vi "remove no error text from control.vi"(11 "vis":refnum<vi>[](array[refnum])) -> (0 "error report":errorcluster[](array[cluster]))   [LabVIEW 2013, in "cosmetic changes.lvclass"]
uses:
  cosmetic changes.lvclass
  <vilib>/Utility/VariantDataType/VariantType.lvlib
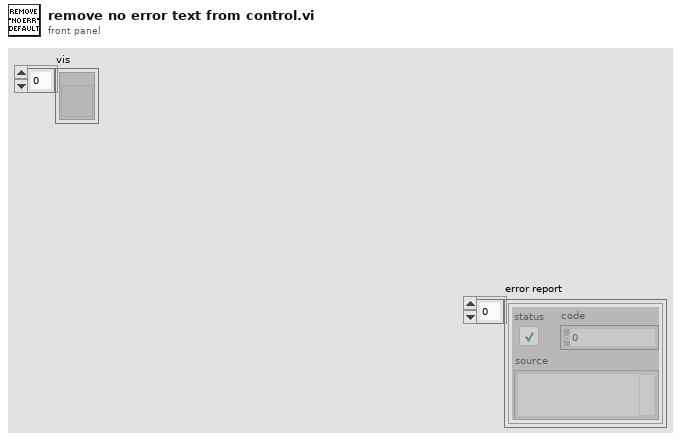
[diagram p1: front panel]
types:
  T1 = typedef "VariantType.lvlib/Type.ctl" = enum8{"Invalid Type", "Void", "I8", "I16", "I32", "I64", "U8", "U16", "U32", "U64", "Single Float", "Double Float", "Extended Float", "Single Complex", "Double Complex", "Extended Complex", "Enum U8", "Enum U16", "Enum U32", "Enum U64", "Single Float With Unit", "Double Float With Unit", "Extended Float With Unit", "Single Complex with Unit", "Double Complex with Unit", "Extended Complex with Unit", "Boolean", "String", "Path", "Picture", "Tag", "Array", "Cluster", "Variant", "LV Variant", "Waveform", "Timestamp", "Digital Waveform", "Digital Data", "ExpressData", "Refnum", "External Data", "VI", "Poly VI", "LabVIEW Class Instance", "Fixed Point"}
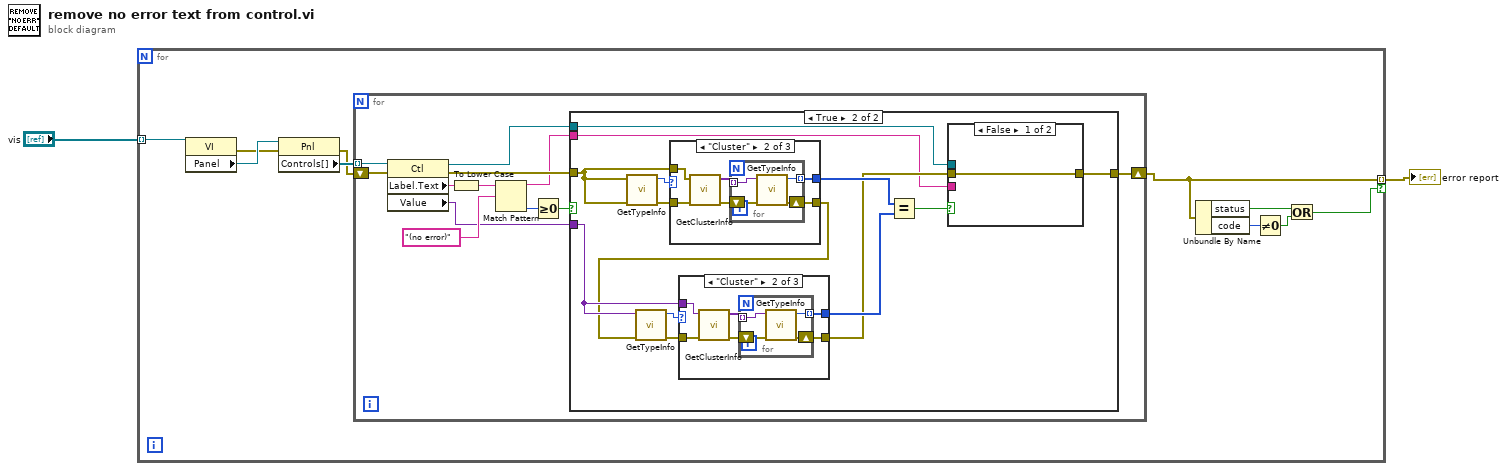
[diagram p0: block diagram]
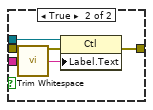
[diagram p3: hidden frame]
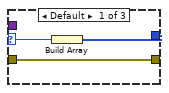
[diagram p4: hidden frame]
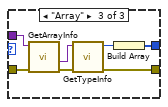
[diagram p5: hidden frame]
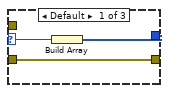
[diagram p6: hidden frame]
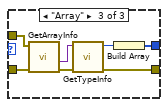
[diagram p7: hidden frame]
diagram:
  n1 = for {
    tunnel: "vis" -> [w8] mode=indexing
    tunnel: [w4] -> w1 mode=indexing if=w3
    n2 = property class="VI"(reference=w8) -> (error out=w11:errorcluster, "Panel"=w12:refnum<vi>)  [unwired: 1 in, 1 out]
    n3 = property class="Pnl"(reference=w12, error in=w11) -> (error out=w9:errorcluster, "Controls[]"=w10:refnum<vi>[])  [unwired: 1 out]
    n4 = for {
      tunnel: w10 -> [w24] mode=indexing
      shift-right: [w15] -> w4
      shift-left: w9 -> [w23]
      n5 = property class="Ctl"(reference=w24, error in=w23) -> (reference out=w14:refnum<vi>, error out=w16:errorcluster, "Label.Text"=w22:string, "Value"=w17:variant)
      n6 = To Lower Case(string=w22) -> (all lower case string=w21:string)
      n7 = Match Pattern(string=w21, regular expression="(no error)") -> (before substring=w13:string, offset past match=w19:i32)  [unwired: 1 in, 2 out]
      n8 = Greater Or Equal To 0?(x=w19) -> (x >= 0?=w18:bool)
      n9 = case shown="True" w18 {
        tunnel: w17 -> [_ w34]
        tunnel: w16 -> [w25 w37]
        tunnel: [w25 w29] -> w15
        tunnel: w14 -> [_ w28]
        tunnel: w13 -> [_ w27]
        frame False {
        }
        frame True {
          n10 = call <vilib>:"GetTypeInfo.vi"("error in (no error)"=w37, "Variant"=w37) -> ("error out"=w38:errorcluster, "Type Enum"=w39:T1)  [unwired: 5 in, 3 out]
          n11 = case shown="\"Cluster\"" w39 {
            selector: w39 -> [w68 _ _]
            tunnel: w37 -> [_ w74 w85]
            tunnel: [w67 w72 w82] -> w32
            tunnel: w38 -> [w66 w71 w80]
            tunnel: [w66 w69 w79] -> w33
            frame Default {
              n12 = Build Array(w68) -> (w67:T1[])
            }
            frame "Cluster" {
              n13 = call <vilib>:"GetClusterInfo.vi"("error in (no error)"=w71, "Variant"=w74) -> ("error out"=w70:errorcluster, "Cluster Elements"=w73:variant[])  [unwired: 8 in]
              n14 = for {
                tunnel: w73 -> [w78] mode=indexing
                tunnel: [w77] -> w72 mode=indexing
                shift-right: [w76] -> w69
                shift-left: w70 -> [w75]
                n15 = call <vilib>:"GetTypeInfo.vi"("error in (no error)"=w75, "Variant"=w78) -> ("error out"=w76:errorcluster, "Type Enum"=w77:T1)  [unwired: 5 in, 3 out]
              }
            }
            frame "Array" {
              n16 = call <vilib>:"GetArrayInfo.vi"("error in (no error)"=w80, "Variant"=w85) -> ("error out"=w81:errorcluster, "ArrayElement"=w84:variant)  [unwired: 6 in, 2 out]
              n17 = call <vilib>:"GetTypeInfo.vi"("error in (no error)"=w81, "Variant"=w84) -> ("error out"=w79:errorcluster, "Type Enum"=w83:T1)  [unwired: 5 in, 3 out]
              n18 = Build Array(w83) -> (w82:T1[])
            }
          }
          n19 = call <vilib>:"GetTypeInfo.vi"("error in (no error)"=w33, "Variant"=w34) -> ("error out"=w36:errorcluster, "Type Enum"=w35:T1)  [unwired: 5 in, 3 out]
          n20 = case shown="\"Cluster\"" w35 {
            selector: w35 -> [w48 _ _]
            tunnel: w34 -> [_ w54 w65]
            tunnel: [w47 w52 w62] -> w31
            tunnel: w36 -> [w46 w51 w60]
            tunnel: [w46 w49 w59] -> w30
            frame Default {
              n21 = Build Array(w48) -> (w47:T1[])
            }
            frame "Cluster" {
              n22 = call <vilib>:"GetClusterInfo.vi"("error in (no error)"=w51, "Variant"=w54) -> ("error out"=w50:errorcluster, "Cluster Elements"=w53:variant[])  [unwired: 8 in]
              n23 = for {
                tunnel: w53 -> [w58] mode=indexing
                tunnel: [w57] -> w52 mode=indexing
                shift-right: [w56] -> w49
                shift-left: w50 -> [w55]
                n24 = call <vilib>:"GetTypeInfo.vi"("error in (no error)"=w55, "Variant"=w58) -> ("error out"=w56:errorcluster, "Type Enum"=w57:T1)  [unwired: 5 in, 3 out]
              }
            }
            frame "Array" {
              n25 = call <vilib>:"GetArrayInfo.vi"("error in (no error)"=w60, "Variant"=w65) -> ("error out"=w61:errorcluster, "ArrayElement"=w64:variant)  [unwired: 6 in, 2 out]
              n26 = call <vilib>:"GetTypeInfo.vi"("error in (no error)"=w61, "Variant"=w64) -> ("error out"=w59:errorcluster, "Type Enum"=w63:T1)  [unwired: 5 in, 3 out]
              n27 = Build Array(w63) -> (w62:T1[])
            }
          }
          n28 = Equal?(x=w32, y=w31) -> (x = y?=w26:bool)
          n29 = case shown="False" w26 {
            tunnel: w30 -> [w40 w45]
            tunnel: [w40 w44] -> w29
            tunnel: w28 -> [_ w43]
            tunnel: w27 -> [_ w41]
            frame False {
            }
            frame True {
              n30 = call <vilib>:"Trim Whitespace.vi"("string"=w41) -> ("trimmed string"=w42:string)  [unwired: 1 in]
              n31 = property class="Ctl"(reference=w43, error in=w45, "Label.Text"=w42) -> (error out=w44:errorcluster)  [unwired: 1 out]
            }
          }
        }
      }
    }
    n32 = Unbundle By Name(w4) -> ("status"=w5:bool, "code"=w6:i32)
    n33 = Not Equal To 0?(x=w6) -> (x != 0?=w7:bool)
    n34 = Or(x=w5, y=w7) -> (x .or. y?=w3:bool)
  }
  "error report" <- w1
